vi "Get Transfer Offsets.vi"(8 "error in (no error)":errorcluster, 10 "Transfer":refnum<class "Transfer.lvclass">, 11 "Transfer Group in":refnum<class "Transfer Group.lvclass">) -> (0 "error out":errorcluster, 1 "group string buffer offset":u64 format="%d bytes", 2 "group engine buffer offset":u64 format="%d bytes", 3 "Transfer Group out":refnum<class "Transfer Group.lvclass">, 4 "Transfer found?":bool)   [LabVIEW 2017, in "DSF Core.lvlib" / "Transfer Group.lvclass"]
uses:
  Transfer Group.lvclass
  Transfer/Transfer.lvclass
  Transfer Group.lvclass/Transfer Group.ctl
  Buffers/Buffers.lvclass
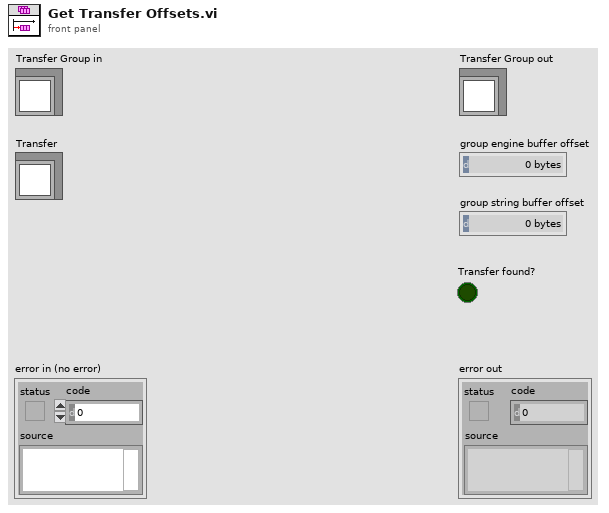
[diagram p1: front panel]
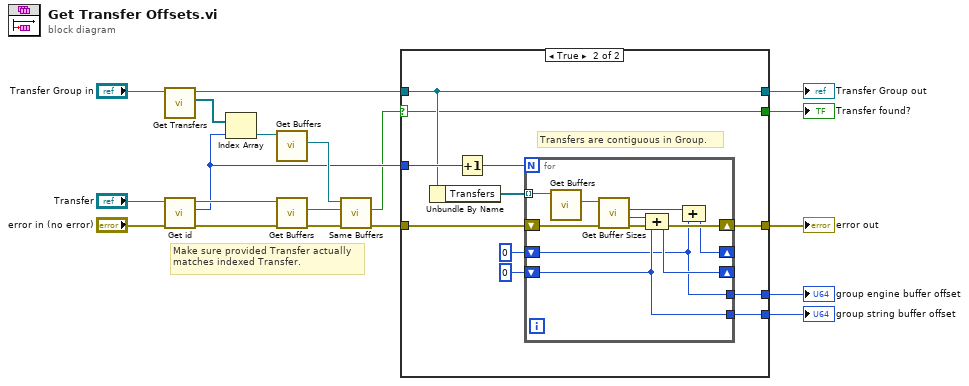
[diagram p0: block diagram]
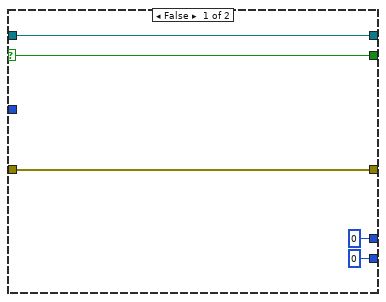
[diagram p2: hidden frame]
diagram:
  # "Make sure provided Transfer actually matches indexed Transfer."
  n1 = call "Get Transfers.vi"("Transfer Group in"="Transfer Group in") -> ("Transfers"=w8:refnum<class "Transfer.lvclass">[], "Transfer Group out"=w13:refnum<class "Transfer Group.lvclass">)  [unwired: 9 in]
  n2 = call "Get id.vi"("Transfer in"="Transfer") -> ("id"=w5:i32, "Transfer out"=w15:refnum<class "Transfer.lvclass">)  [unwired: 9 in]
  n3 = Index Array(array=w8, index=w5) -> (element=w14:refnum<class "Transfer.lvclass">)
  n4 = call "Get Buffers.vi"("Transfer in"=w14) -> ("Buffers"=w6:refnum<class "Buffers.lvclass">)  [unwired: 9 in, 1 out]
  n5 = call "Get Buffers.vi"("Transfer in"=w15) -> ("Buffers"=w7:refnum<class "Buffers.lvclass">)  [unwired: 9 in, 1 out]
  n6 = call "Same Buffers.vi"("error in (no error)"="error in (no error)", "Buffers 2"=w7, "Buffers 1"=w6) -> ("error out"=w9:errorcluster, "same buffers?"=w2:bool)  [unwired: 7 in]
  n7 = case shown="True" w2 {
    selector: w2 -> [w18 w23]
    tunnel: w13 -> [w22 w24]
    tunnel: [w22 w24] -> w12
    tunnel: w9 -> [w21 w31]
    tunnel: [w21 w30] -> w11
    tunnel: w5 -> [_ w27]
    tunnel: [u64 0 ("engine buffer size") w28] -> w3
    tunnel: [u64 0 ("engine buffer size") w29] -> w4
    tunnel: [w18 w23] -> w1
    frame False {
    }
    frame True {
      # "Transfers are contiguous in Group."
      n8 = Unbundle By Name(w24) -> ("Transfers"=w32:refnum<class "Transfer.lvclass">[])
      n9 = Increment(x=w27) -> (x+1=w33:i32)
      n10 = for {
        N: w33 -> [_]
        tunnel: w32 -> [w43] mode=indexing
        shift-right: [w36] -> _
        shift-left: u64 0 ("engine buffer size") -> [w34]
        shift-right: [w41] -> _
        shift-left: u64 0 ("engine buffer size") -> [w35]
        shift-right: [w40] -> w30
        shift-left: w31 -> [w39]
        tunnel: [w35] -> w29
        tunnel: [w34] -> w28
        n11 = call "Get Buffers.vi"("Transfer in"=w43) -> ("Buffers"=w42:refnum<class "Buffers.lvclass">)  [unwired: 9 in, 1 out]
        n12 = call "Get Buffer Sizes.vi"("error in (no error)"=w39, "Buffers in"=w42) -> ("error out"=w40:errorcluster, "string buffer size"=w38:u64, "engine buffer size"=w37:u64)  [unwired: 6 in, 1 out]
        n13 = Compound Arithmetic op=ADD(w38, w35) -> (w41:u64)
        n14 = Compound Arithmetic op=ADD(w37, w34) -> (w36:u64)
      }
    }
  }
  "error out" <- w11
  "Transfer Group out" <- w12
  "group engine buffer offset" <- w3
  "group string buffer offset" <- w4
  "Transfer found?" <- w1
